vi "test for set channel.vi"() -> ()   [LabVIEW 2013]
uses:
  Set Channels.lvlib
  <vilib>/NI Veristand/Execution/Workspace/NI_VS Workspace ExecutionAPI.lvlib
  <vilib>/NI Veristand/Execution/Workspace/NI VeriStand - Get Single Channel Value.vi
  <vilib>/NI Veristand/Execution/Workspace/NI VeriStand - Set Single Channel Value.vi
panel:
  in  "Blocking?":bool
  out "Value":dbl
  in  "newVal":dbl format="%#_13g"
  in  "name":string="Targets/Controller/Simulation Models/Models/Engine Demo/Inports/command_EngineOn"
  out "error out":errorcluster
  out "Report Text":string
  # "Deploy system before running!"
  # "Also, disable TestStand calls in the VI!"
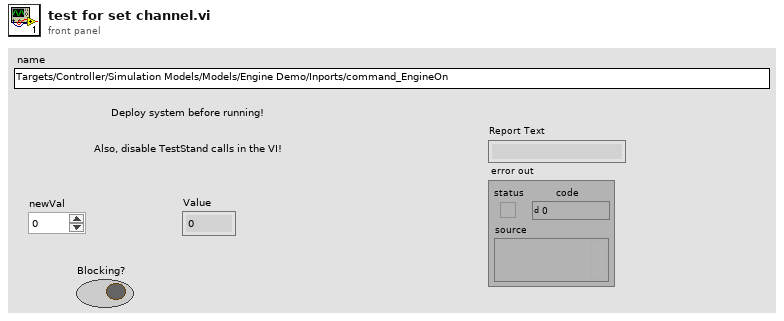
[diagram p1: front panel]
types:
  T1 = typedef "NI_VS Workspace ExecutionAPI.lvlib/WorkspaceAPI.ctl" = refnum<k24>
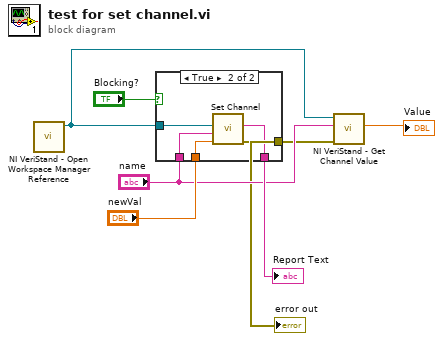
[diagram p0: block diagram]
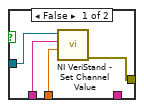
[diagram p2: hidden frame]
diagram:
  n1 = call <vilib>:"NI VeriStand - Open Workspace Manager Reference.vi"() -> ("WorkspaceManager"=w5:T1)  [unwired: 10 in, 1 out]
  n2 = case shown="True" "Blocking?" {
    tunnel: "newVal" -> [w10 w16]
    tunnel: [_ w15] -> w6
    tunnel: w5 -> [w9 w14]
    tunnel: "name" -> [w11 w13]
    tunnel: [w8 w12] -> w2
    frame False {
      n3 = call-poly <vilib>:"NI VeriStand - Set Channel Value.vi"("Value"=w10, "Channel"=w11, "WorkspaceManager in"=w9) -> ("error out"=w8:errorcluster)  [unwired: 7 in, 1 out]
    }
    frame True {
      n4 = call "Set Channel.vi"("newVal"=w16, "name"=w13, "Gateway IP Address (\"\": localhost)"=w14) -> ("error out"=w12:errorcluster, "Report Text"=w15:string)  [unwired: 6 in, 1 out]
    }
  }
  "Report Text" <- w6
  "error out" <- w2
  n5 = call-poly <vilib>:"NI VeriStand - Get Channel Value.vi"("error in (no error)"=w2, "Channel"="name", "WorkspaceManager in"=w5) -> ("Value"=→"Value":dbl)  [unwired: 6 in, 2 out]
